vi "close.vi"(8 "error in (no error)":errorcluster, 11 "Item in":refnum<class "Item.lvclass">) -> (0 "error out":errorcluster)   [LabVIEW 2020, in "toml_edit.lvlib" / "Item.lvclass"]
uses:
  Item.lvclass
  Item.lvclass/Item.ctl
  dragon_toml_64.dll
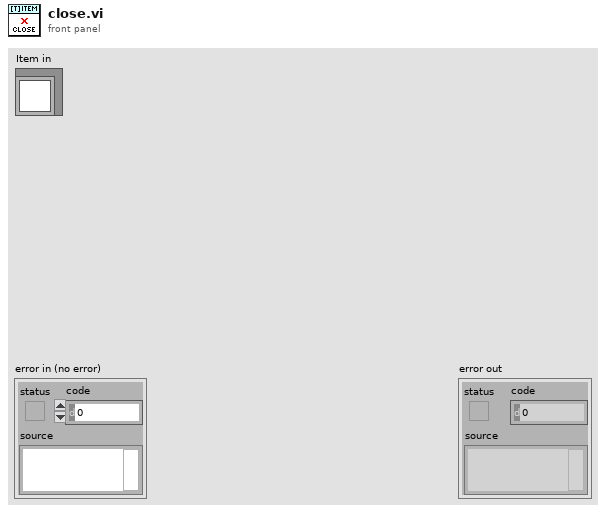
[diagram p1: front panel]
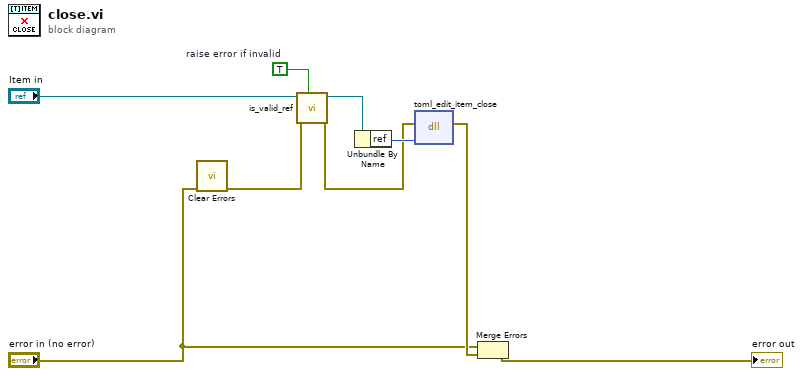
[diagram p0: block diagram]
diagram:
  w1 = TRUE  # raise error if invalid
  n1 = call <vilib>:"Clear Errors.vi"("error in (no error)"="error in (no error)") -> ("error out"=w3:errorcluster)  [unwired: 5 in, 1 out]
  n2 = call-dynamic "is_valid_ref.vi"("raise error if invalid? (False)"=w1, "error in (no error)"=w3, "Item in"="Item in") -> ("error out"=w2:errorcluster, "Item out"=w4:refnum<class "Item.lvclass">)  [unwired: 6 in, 1 out]
  n3 = Unbundle By Name(w4) -> ("ref"=w8:u64)
  n4 = dll-call lib="C:/Projects/labview-project-load-tools/source/submodules/toml-edit-labview/lv_src/dragon_toml_*.*" fn="toml_edit_item_close"(error in=w2, "item_ref"=w8) -> (error out=w9:errorcluster)  [unwired: 4 in, 1 out]
  n5 = Merge Errors("error in (no error)", w9) -> (→"error out":errorcluster)
